vi "Extract Samples from AVI.vi"(8 "error in (no error)":errorcluster, 11 "AVI Path":path) -> (0 "error out":errorcluster, 3 "Samples":dbl[][](array[numeric]))   [LabVIEW 2013]
uses:
  <vilib>/vision/NI_Vision_Development_Module.lvlib
panel:
  out "Number of Samples":dbl
  in  "ROI Height":i32=100
  in  "ROI Width":i32=100
  in  "dy":i32=75
  in  "dx":i32=75
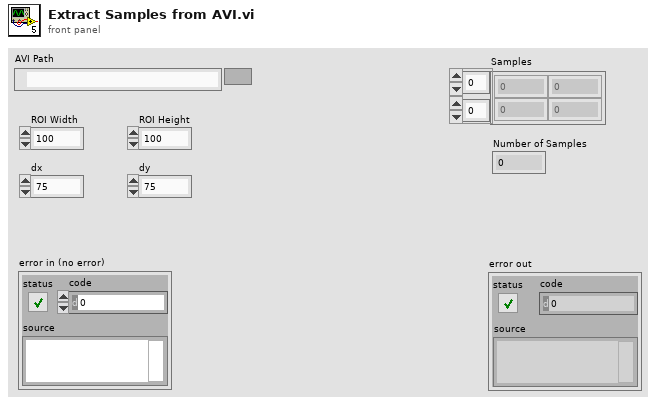
[diagram p1: front panel]
types:
  T1 = typedef "IMAQ Image.ctl" = refnum<image>
  T2 = typedef "IMAQ Rectangle" = cluster{"Left":i32, "Top":i32, "Right":i32, "Bottom":i32, "Rotation":dbl}
  T3 = typedef "Image Type" = u32
  T4 = typedef "ROI Descriptor" = cluster{"Global Rectangle":i32[], "Contours":cluster{"ID":enum32{"External", "Internal"}, "Type":u32, "Coordinates":i32[]}[]}
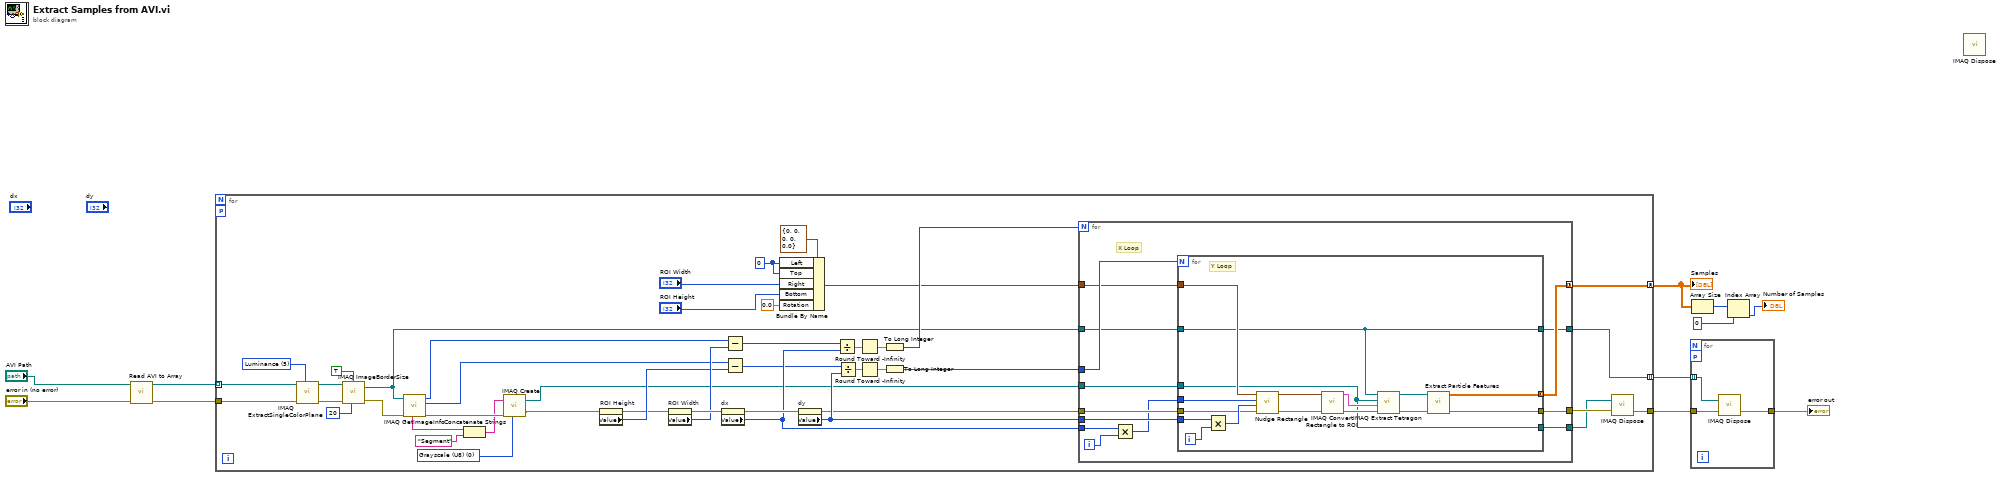
[diagram p0: block diagram]
diagram:
  n1 = call "Read AVI to Array.vi"("Error in (no error)"="error in (no error)", "AVI Path"="AVI Path") -> ("Error out"=w9:errorcluster, "Image Array"=w8:T1[])  [unwired: 7 in, 1 out]
  n2 = for {
    tunnel: w9 -> [w56]
    tunnel: w8 -> [w55] mode=indexing
    workers-P: _ -> [_]
    tunnel: [w14] -> w6
    tunnel: [w13] -> w4 mode=concatenating
    tunnel: [w12] -> w5 mode=indexing
    w23 = 0 ("Left")
    w49 = T3 0 items=["Grayscale (U8)", "Grayscale (I16)", "Grayscale (SGL)", "Complex (CSG)", "RGB (U32)", "HSL (U32)", "RGB (U64)", "Grayscale (U16)"] ("Image Type")
    w54 = 5 items=["Red", "Green", "Blue", "Hue", "Saturation", "Luminance", "Value", "Intensity"] ("Color Plane")
    n3 = call "IMAQ ExtractSingleColorPlane"("Color Plane"=w54, "error in (no error)"=w56, "Image Src"=w55) -> ("error out"=w46:errorcluster, "Image Dst Out"=w45:T1)  [unwired: 7 in]
    n4 = call "IMAQ ImageBorderSize"("Get/Set Status? (Set)"=TRUE, "Image"=w45, "Image border size in"=20 ("Border Size"), "error in (no error)"=w46) -> ("Image Out"=w18:T1, "error out"=w44:errorcluster)  [unwired: 1 out]
    n5 = call "IMAQ GetImageInfo"("error in (no error)"=w44, "Image"=w18) -> ("error out"=w51:errorcluster, "Y Resolution"=w20:i32, "X Resolution"=w21:i32, "Image Name"=w53:string)  [unwired: 2 in, 4 out]
    n6 = Concatenate Strings(w53, "Segment" ("string")) -> (w50:string)
    n7 = call "IMAQ Create"("Image Name"=w50, "Image Type"=w49, "error in (no error)"=w51) -> ("New Image"=w17:T1, "error out"=w19:errorcluster)  [unwired: 2 in]
    n8 = property on="ROI Height" class="DigNum (strict)"(error in=w19) -> (error out=w25:errorcluster, "Value"=w30:i32)  [unwired: 1 in, 1 out]
    n9 = property on="ROI Width" class="DigNum (strict)"(error in=w25) -> (error out=w39:errorcluster, "Value"=w31:i32)  [unwired: 1 in, 1 out]
    n10 = property on="dx" class="DigNum (strict)"(error in=w39) -> (error out=w41:errorcluster, "Value"=w40:i32)  [unwired: 1 in, 1 out]
    n11 = Subtract(x=w21, y=w31) -> (x-y=w32:i32)
    n12 = Subtract(x=w20, y=w30) -> (x-y=w33:i32)
    n13 = Bundle By Name(cluster=T2 {"Left"=0, "Top"=0, "Right"=0, "Bottom"=0, "Rotation"=0.0} ("Rectangle"), "Left"=w23, "Top"=w23, "Right"="ROI Width", "Bottom"="ROI Height", "Rotation"=0.0) -> (w37:T2)
    n14 = property on="dy" class="DigNum (strict)"(error in=w41) -> (error out=w42:errorcluster, "Value"=w43:i32)  [unwired: 1 in, 1 out]
    n15 = Divide(x=w32, y=w40) -> (x/y=w26:dbl)
    n16 = Divide(x=w33, y=w43) -> (x/y=w28:dbl)
    n17 = Round Toward -Infinity(1:w26) -> (0:w27:dbl)
    n18 = Round Toward -Infinity(1:w28) -> (0:w29:dbl)
    n19 = To Long Integer(number=w27) -> (32bit integer=w38:i32)
    n20 = To Long Integer(number=w29) -> (32bit integer=w36:i32)
    n21 = for {
      N: w38 -> [_]
      tunnel: w36 -> [w69]
      tunnel: w40 -> [w68]
      tunnel: w43 -> [w67]
      tunnel: w42 -> [w66]
      tunnel: w37 -> [w65]
      tunnel: w18 -> [w62]
      tunnel: w17 -> [w61]
      tunnel: [w60] -> w15
      tunnel: [w59] -> w13 mode=concatenating
      tunnel: [w58] -> w16
      tunnel: [w57] -> w12
      i -> [w63]
      # "X Loop"
      n22 = Multiply(x=w68, y=w63) -> (x*y=w64:i32)
      n23 = for {
        N: w69 -> [_]
        tunnel: w67 -> [w85]
        tunnel: w66 -> [w79]
        tunnel: w65 -> [w83]
        tunnel: w64 -> [w81]
        tunnel: w62 -> [w70]
        tunnel: w61 -> [w71]
        tunnel: [w73] -> w58
        tunnel: [w72] -> w59 mode=concatenating
        tunnel: [w71] -> w60
        tunnel: [w70] -> w57
        i -> [w84]
        # "Y Loop"
        n24 = Multiply(x=w85, y=w84) -> (x*y=w80:i32)
        n25 = call "Nudge Rectangle.vi"("error in (no error)"=w79, "dy"=w80, "dx"=w81, "Rectangle"=w83) -> ("error out"=w78:errorcluster, "Nudged Rectangle"=w82:T2)  [unwired: 6 in]
        n26 = call "IMAQ Convert Rectangle to ROI"("error in (no error)"=w78, "Rectangle"=w82) -> ("error out"=w77:errorcluster, "ROI Descriptor"=w76:T4)  [unwired: 7 in]
        n27 = call-poly "IMAQ Extract Tetragon"("error in (no error)"=w77, "ROI Descriptor"=w76, "Image Dst"=w71, "Image Src"=w70) -> ("error out"=w75:errorcluster, "Image Dst Out"=w74:T1)  [unwired: 6 in]
        n28 = call "Extract Particle Features.vi"("error in (no error)"=w75, "Segment Image"=w74) -> ("error out"=w73:errorcluster, "Particle Features"=w72:dbl[][])  [unwired: 8 in]
      }
    }
    n29 = call "IMAQ Dispose"("Image"=w15, "error in (no error)"=w16) -> ("error out"=w14:errorcluster)  [unwired: 4 in]
  }
  "Samples" <- w4
  n30 = for {
    tunnel: w5 -> [w86] mode=indexing
    workers-P: _ -> [_]
    tunnel: w6 -> [w87]
    tunnel: [w88] -> w7
    n31 = call "IMAQ Dispose"("Image"=w86, "error in (no error)"=w87) -> ("error out"=w88:errorcluster)  [unwired: 4 in]
  }
  "error out" <- w7
  n32 = Array Size(array=w4) -> (size(s)=w3:i32[])
  n33 = Index Array(array=w3, index=0) -> (element=→"Number of Samples":i32)
  n34 = call "IMAQ Dispose"() -> ()  [unwired: 6 in, 1 out]
